vi "Compare_Project_Cache.vi"(8 "error in (no error)":errorcluster, 11 "AB_Build in":refnum<class "AB_Build.lvclass">) -> (0 "error out":errorcluster, 2 "valid?":bool, 3 "AB_Build out":refnum<class "AB_Build.lvclass">)   [LabVIEW 2020, in "AB_Build.lvclass"]
uses:
  <vilib>/AppBuilder/AB_Classes/Build/AB_Build.lvclass
  <vilib>/AppBuilder/AB_Classes/Build/AB_Build.lvclass/AB_Build.ctl
  <vilib>/AppBuilder/AB_Classes/PreviewCache/PreviewCache.lvclass
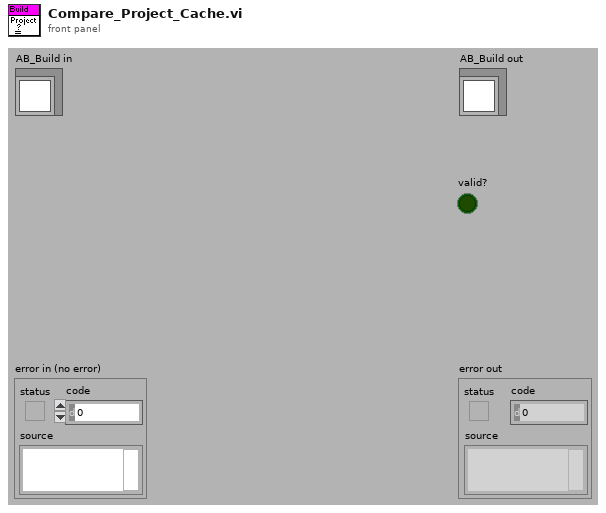
[diagram p1: front panel]
types:
  T1 = typedef "ItemRef.ctl" = u64
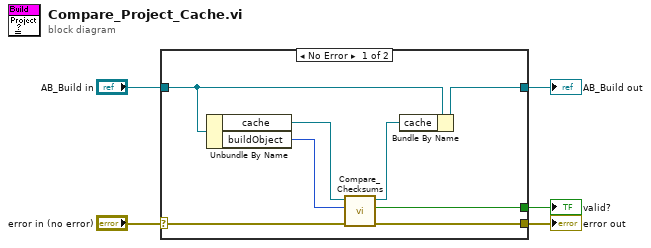
[diagram p0: block diagram]
diagram:
  n1 = case shown="No Error" "error in (no error)" {
    selector: "error in (no error)" -> [w10 w15]
    tunnel: [w9 w15] -> w4
    tunnel: [w7 w14] -> w2
    tunnel: "AB_Build in" -> [w8 w14]
    tunnel: [w11 _] -> w1
    frame No Error {
      n2 = Unbundle By Name(w8) -> ("cache"=w13:refnum<class "PreviewCache.lvclass">, "buildObject"=w12:T1)
      n3 = call <vilib>:"Compare_Checksums.vi"("error in (no error)"=w10, "build object"=w12, "PreviewCache"=w13) -> ("error out"=w9:errorcluster, "valid?"=w11:bool, "PreviewCache out"=w6:refnum<class "PreviewCache.lvclass">)  [unwired: 6 in]
      n4 = Bundle By Name(cluster=w8, "cache"=w6) -> (w7:refnum<class "AB_Build.lvclass">)
    }
    frame Error {
    }
  }
  "error out" <- w4
  "AB_Build out" <- w2
  "valid?" <- w1
